vi "Setup Motors.vi"   [LabVIEW 2014]
uses:
  <vilib>/Rock Robotics/SystemInterfaces/DIO/FPGA_DIOPWMChannel.ctl
  <vilib>/Rock Robotics/WPI/Joystick/WPI_JoystickDeviceEnum.ctl
  <vilib>/Rock Robotics/SystemInterfaces/Typedef/FPGA_TypedefDigitalModule.ctl
  <vilib>/Rock Robotics/SystemInterfaces/Typedef/FPGA_TypedefAnalogModule.ctl
  <vilib>/Rock Robotics/SystemInterfaces/AI/FPGA_AIChannel.ctl
  <vilib>/Rock Robotics/WPI/SafetyOutput/WPI_SafetyOutputConfigMenu.ctl
  <vilib>/Rock Robotics/WPI/Solenoid/WPI_SolenoidChannel.ctl
  <vilib>/Rock Robotics/SystemInterfaces/AI/FPGA_AIGyroChannel.ctl
  <vilib>/Rock Robotics/SystemInterfaces/Typedef/FPGA_TypedefAnalogModuleForGyro.ctl
  <vilib>/Rock Robotics/SystemInterfaces/DIO/FPGA_DIOChannel.ctl
  NavX Code/navX-MXP Library/COMMON/TypeDefs/Value TypeDefs/navX Interface Protocol.ctl
  <vilib>/Rock Robotics/SystemInterfaces/spilib/spi_bus.ctl
  <vilib>/Rock Robotics/SystemInterfaces/i2clib/i2c_bus.ctl
  NavX Code/navX-MXP Library/COMMON/TypeDefs/Value TypeDefs/navX Update Rate.ctl
  <vilib>/Rock Robotics/WPI/MotorControl/WPI_MotorControlOpen Jaguar.vi
  <vilib>/Rock Robotics/WPI/MotorControl/WPI_MotorControlOpen Talon.vi
  <vilib>/Rock Robotics/WPI/Solenoid/WPI_SolenoidOpenSingle.vi
  <vilib>/Rock Robotics/WPI/Switch/WPI_SwitchOpenLimit.vi
  <vilib>/Rock Robotics/WPI/Counter/WPI_CounterDigitalInputToDigitalSource.vi
  <vilib>/Rock Robotics/WPI/Counter/WPI_CounterOpen UpDown Mode.vi
  Global Variables.vi
  NavX Code/navX-MXP Library/navX-MXP IMU.lvlib
types:
  T1 = typedef "FPGA_DIOChannel.ctl" = enum8{"DIO 0", "DIO 1", "DIO 2", "DIO 3", "DIO 4", "DIO 5", "DIO 6", "DIO 7", "DIO 8", "DIO 9", "DIO MXP 0", "DIO MXP 1", "DIO MXP 2", "DIO MXP 3", "DIO MXP 4", "DIO MXP 5", "DIO MXP 6", "DIO MXP 7", "DIO MXP 8", "DIO MXP 9", "DIO MXP 10", "DIO MXP 11", "DIO MXP 12", "DIO MXP 13", "DIO MXP 14", "DIO MXP 15", "Invalid"}
  T2 = typedef "navX-MXP IMU.lvlib/navX Update Rate.ctl" = u8
  T3 = typedef "i2c_bus.ctl" = enum16{"I2C On-Board", "I2C MXP", "Invalid"}
  T4 = typedef "spi_bus.ctl" = enum16{"SPI On-Board, CS0", "SPI On-Board, CS1", "SPI On-Board, CS2", "SPI On-Board, CS3", "SPI MXP", "Invalid"}
  T5 = typedef "navX-MXP IMU.lvlib/navX Interface Protocol.ctl" = enum16{"SPI", "I2C"}
  T6 = typedef "WPI_SafetyOutputConfigMenu.ctl" = enum16{"Enable", "Disable"}
  T7 = typedef "FPGA_TypedefDigitalModule.ctl" = enum16{"Controller 1"}
  T8 = typedef "FPGA_TypedefAnalogModuleForGyro.ctl" = enum16{"Controller 1"}
  T9 = typedef "FPGA_AIGyroChannel.ctl" = enum8{"AI 0", "AI 1", "Invalid"}
  T10 = typedef "WPI_SolenoidChannel.ctl" = enum8{"Solenoid 0", "Solenoid 1", "Solenoid 2", "Solenoid 3", "Solenoid 4", "Solenoid 5", "Solenoid 6", "Solenoid 7", "Invalid"}
  T11 = typedef "FPGA_DIOPWMChannel.ctl" = enum8{"PWM 0", "PWM 1", "PWM 2", "PWM 3", "PWM 4", "PWM 5", "PWM 6", "PWM 7", "PWM 8", "PWM 9", "PWM MXP 0", "PWM MXP 1", "PWM MXP 2", "PWM MXP 3", "PWM MXP 4", "PWM MXP 5", "PWM MXP 6", "PWM MXP 7", "PWM MXP 8", "PWM MXP 9", "Invalid"}
  T12 = typedef "FPGA_AIChannel.ctl" = enum8{"AI 0", "AI 1", "AI 2", "AI 3", "AI MXP 0", "AI MXP 1", "AI MXP 2", "AI MXP 3", "Invalid"}
  T13 = typedef "FPGA_TypedefAnalogModule.ctl" = enum16{"Controller 1"}
  T14 = typedef "WPI_JoystickDeviceEnum.ctl" = enum16{"USB 0", "USB 1", "USB 2", "USB 3", "USB 4", "USB 5"}
  T15 = typedef "WPI_MotorControlDeviceRef.ctl" = cluster{"DeviceStatus":errorcluster, "Type":T16, "PWM":cluster{"Controller":T7, "PWM Channel":T11, "DeadBand":T17}, "CAN":cluster{"Device Number":u8, "Control Mode":T18, "Semaphore":T19, "Max Vout":dbl, "TalonSRX Control Mode":T20}, "Invert":bool, "TransformRef":T21, "InvTransformRef":T21}
  T16 = typedef "WPI_MotorControlType.ctl" = enum16{"PWM", "CAN", "CANTalonSRX"}
  T17 = typedef "WPI_PWMDeadband.ctl" = cluster{"Name":string, "maxPositivePwm":i32, "minPositivePwm":i32, "centerPwm":i32, "maxNegativePwm":i32, "minNegativePwm":i32, "angularRange":u16}
  T18 = typedef "WPI_CANJaguar_ControlMode.ctl" = enum8{"Percent VBus", "Current", "Speed", "Position", "Voltage"}
  T19 = typedef "Semaphore RefNum" = refnum<k1>
  T20 = typedef "WPI_CANTalonSRX_APIControlMode.ctl" = enum8{"Percent VBus", "Speed", "Position", "Slave", "Unchanged / Invalid"}
  T21 = typedef "WPI_PWMTransform_ConPane.ctl" = refnum<vi>
  T22 = typedef "WPI_GyroDevRef.ctl" = cluster{"DevStatus":errorcluster, "Analog Module":T13, "Analog Channel":T12, "Offset":dbl, "Gain (VoltsPerDegree/Second)":dbl}
  T23 = typedef "WPI_SolenoidDevRef.ctl" = cluster{"DevStatus":errorcluster, "Pneumatics Control Module":u8, "Forward Solenoid Channel":T10, "Reverse Solenoid Channel":T10}
  T24 = typedef "WPI_SwitchDevRef.ctl" = cluster{"DevStatus":errorcluster, "DIO Channel":T1, "Controller":T7, "CntIndex":T25, "Normally Closed":bool}
  T25 = typedef "FPGA_CounterCtrSystemIndex.ctl" = enum8{"Ctr 0", "Ctr 1", "Ctr 2", "Ctr 3", "Ctr 4", "Ctr 5", "Ctr 6", "Ctr 7", "Invalid"}
  T26 = typedef "WPI_AnalogChannelDevRef.ctl" = cluster{"DevStatus":errorcluster, "Controller":T13, "Analog Channel":T12}
  T27 = typedef "WPI_DigitalInputDevRef.ctl" = cluster{"DevStatus":errorcluster, "DIO Channel":T1, "Controller":T7}
  T28 = typedef "FPGA_CounterEncoderSourceConvertionLVSourceType.ctl" = cluster{"DevStatus":errorcluster, "AnalogTriggerMode?":bool, "DigitalMode":cluster{"Controller":T7, "DIO Channel":T29}, "AnalogTriggerMode":cluster{"AnalogTriggerIndex":T30, "OutputType":T31}}
  T29 = typedef "FPGA_DIODigitalSourceChannel.ctl" = enum8{"DIO 0", "DIO 1", "DIO 2", "DIO 3", "DIO 4", "DIO 5", "DIO 6", "DIO 7", "DIO 8", "DIO 9", "DIO MXP 0", "DIO MXP 1", "DIO MXP 2", "DIO MXP 3", "DIO MXP 4", "DIO MXP 5", "DIO MXP 6", "DIO MXP 7", "DIO MXP 8", "DIO MXP 9", "DIO MXP 10", "DIO MXP 11", "DIO MXP 12", "DIO MXP 13", "DIO MXP 14", "DIO MXP 15", "Disabled"}
  T30 = typedef "FPGA_AnalogTriggerIndex.ctl" = enum8{"Trig 0", "Trig 1", "Trig 2", "Trig 3", "Trig 4", "Trig 5", "Trig 6", "Trig 7", "Invalid"}
  T31 = typedef "FPGA_AnalogTriggerOutType.ctl" = enum16{"InWindow", "TriggerState", "Rising", "Falling"}
  T32 = typedef "WPI_EncoderDevRef.ctl" = cluster{"DevStatus":errorcluster, "EncoderIndex":T33, "CounterIndex":T25, "DistancePerCount":dbl, "Decoding Type":T34}
  T33 = typedef "FPGA_EncoderIdx.ctl" = enum8{"Enc 0", "Enc 1", "Enc 2", "Enc 3", "Enc 4", "Enc 5", "Enc 6", "Enc 7", "Invalid"}
  T34 = typedef "WPI_EncoderType.ctl" = enum16{"1x", "2x", "4x"}
  T35 = typedef "WPI_CounterDevRef.ctl" = cluster{"DevStatus":errorcluster, "CntIndex":T25}
  T36 = typedef "navX-MXP IMU.lvlib/navX Device TypeDef.ctl" = cluster{"navX Interface Protocol":T5, "navX Interface Protocol TypeDefs":cluster{"SPIDevRef":T37, "I2CDevRef":T38}, "navX System Information":cluster{"Board Information":T39, "Status":T40, "Offsets":T44}, "navX Common Information":cluster{"Update Rate (4Hz-60Hz)":T2, "refnum name":string, "error":errorcluster}}
  T37 = typedef "WPI_SPIDevRef.ctl" = cluster{"DevStatus":errorcluster, "Handle":i32, "Controller":T7, "SPI Bus":T4}
  T38 = typedef "WPI_I2CDevRef.ctl" = cluster{"DevStatus":errorcluster, "Controller":T7, "Device Address":u8, "Handle":i32, "I2C Bus":T3}
  T39 = typedef "navX-MXP IMU.lvlib/navX Board Information.ctl" = cluster{"WhoAmI (50 | 0x32)":u8, "Board Revision":u8, "Firmware Major Version":u8, "Firmware Minor Version":u8}
  T40 = typedef "navX-MXP IMU.lvlib/navX Status Data.ctl" = cluster{"Update Rate Hz":u8, "Accelerometer Full-Scale Range":u8, "Gyro Full-Scale Range":u16, "NAVX_OP_STATUS":T41, "NAVX_CAL_STATUS":T42, "NAVX_SELFTEST_STATUS":u8, "NAVX_SENSOR_STATUS":T43}
  T41 = typedef "navX-MXP IMU.lvlib/navX NAVX_OP_STATUS.ctl" = u8
  T42 = typedef "navX-MXP IMU.lvlib/navX NAVX_CAL_STATUS.ctl" = u8
  T43 = typedef "navX-MXP IMU.lvlib/navX NAVX_SENSOR_STATUS.ctl" = cluster{"MOVING":bool, "YAW_STABLE":bool, "MAG_DISTURBANCE":bool, "ALTITUDE_VALID":bool, "SEALEVEL_PRESS_SET":bool, "FUSED_HEADING_VALID":bool}
  T44 = typedef "navX-MXP IMU.lvlib/navX Offsets Data.ctl" = cluster{"Yaw":dbl, "Quat W":dbl, "Quat X":dbl, "Quat Y":dbl, "Quat Z":dbl}
  T45 = typedef "WPI_JoystickDevRef.ctl" = cluster{"Device":T14}
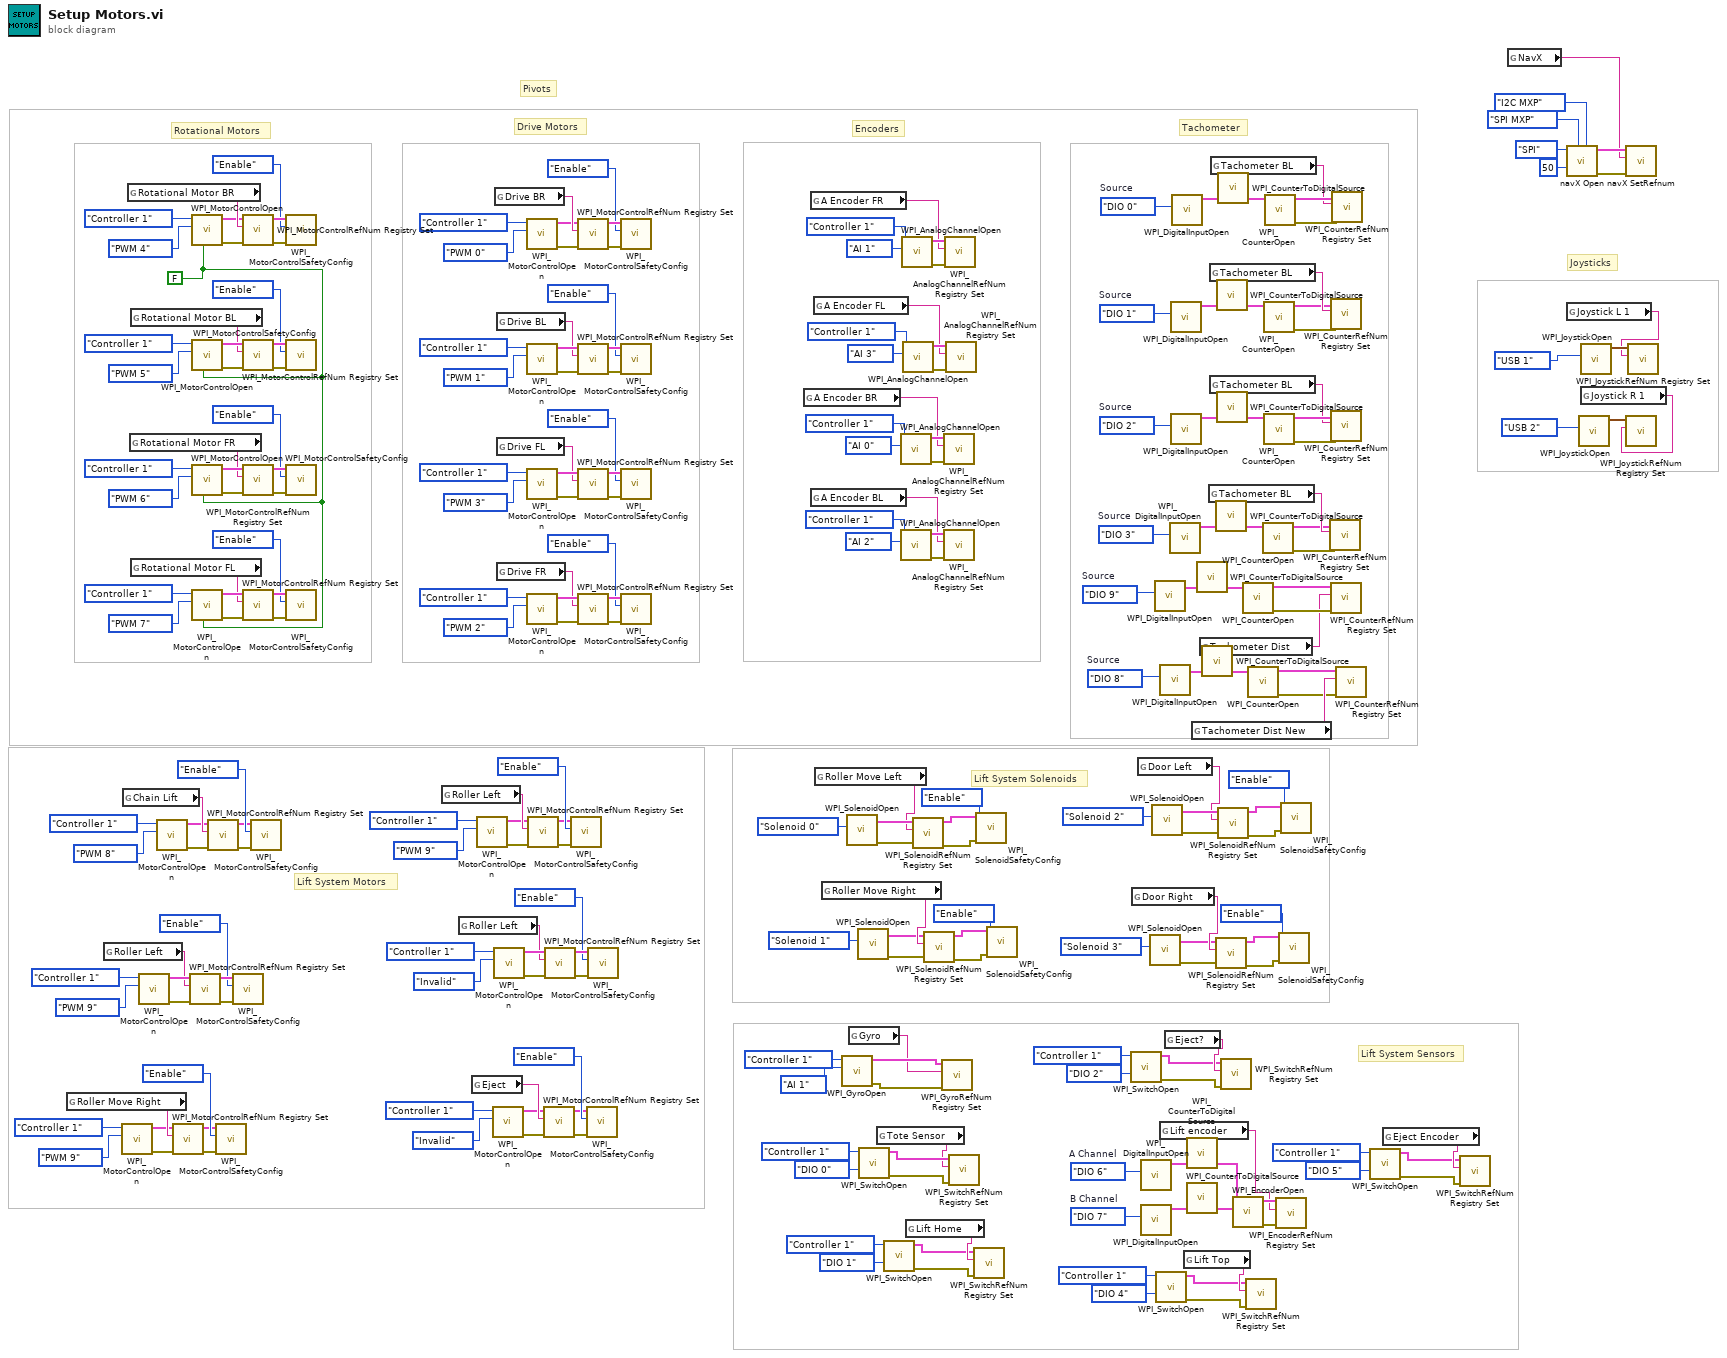
[diagram p0: block diagram]
diagram:
  w4 = FPGA_DIOChannel."DIO 8"  # Source
  w9 = FPGA_DIOChannel."DIO 9"  # Source
  w21 = FPGA_DIOChannel."DIO 3"  # Source
  w30 = FPGA_DIOChannel."DIO 2"  # Source
  w33 = FPGA_DIOChannel."DIO 1"  # Source
  w42 = FPGA_DIOChannel."DIO 0"  # Source
  w44 = FALSE ("Invert")
  w53 = FPGA_DIOChannel."DIO 7"  # B Channel
  w52 = FPGA_DIOChannel."DIO 6"  # A Channel
  # "Tachometer"
  # "Lift System Sensors"
  # "Lift System Solenoids"
  # "Lift System Motors"
  # "Encoders"
  # "Joysticks"
  # "Pivots"
  # "Rotational Motors"
  # "Drive Motors"
  n1 = global read "Global Variables.vi" "Roller Move Right"() -> (w142:string)
  n2 = global read "Global Variables.vi" "Roller Left"() -> (w145:string)
  n3 = call-poly <vilib>:"WPI_MotorControlOpen.vi"("PWM Channel"=FPGA_DIOPWMChannel."PWM 9", "Controller"=FPGA_TypedefDigitalModule."Controller 1") -> ("error out"=w137:errorcluster, "MotorControlDeviceRef"=w136:T15)  [unwired: 8 in]
  n4 = global read "Global Variables.vi" "Chain Lift"() -> (w158:string)
  n5 = global read "Global Variables.vi" "Rotational Motor BR"() -> (w212:string)
  n6 = global read "Global Variables.vi" "Rotational Motor FR"() -> (w186:string)
  n7 = global read "Global Variables.vi" "Rotational Motor BL"() -> (w187:string)
  n8 = global read "Global Variables.vi" "Rotational Motor FL"() -> (w185:string)
  n9 = call-poly <vilib>:"WPI_MotorControlOpen.vi"("PWM Channel"=FPGA_DIOPWMChannel."PWM 9", "Controller"=FPGA_TypedefDigitalModule."Controller 1") -> ("error out"=w150:errorcluster, "MotorControlDeviceRef"=w151:T15)  [unwired: 8 in]
  n10 = call-poly <vilib>:"WPI_MotorControlOpen.vi"("PWM Channel"=FPGA_DIOPWMChannel."PWM 8", "Controller"=FPGA_TypedefDigitalModule."Controller 1") -> ("error out"=w153:errorcluster, "MotorControlDeviceRef"=w152:T15)  [unwired: 8 in]
  n11 = call <vilib>:"WPI_MotorControlRefNum Registry Set.vi"("error in (no error)"=w137, "refnum name"=w142, "MotorControlDevRef"=w136) -> ("error out"=w139:errorcluster, "MotorControlDevRef"=w138:T15)  [unwired: 7 in]
  n12 = call <vilib>:"WPI_MotorControlRefNum Registry Set.vi"("error in (no error)"=w150, "refnum name"=w145, "MotorControlDevRef"=w151) -> ("error out"=w148:errorcluster, "MotorControlDevRef"=w149:T15)  [unwired: 7 in]
  n13 = call-poly <vilib>:"WPI_MotorControlOpen.vi"("Invert"=w44, "PWM Channel"=FPGA_DIOPWMChannel."PWM 4", "Controller"=FPGA_TypedefDigitalModule."Controller 1") -> ("error out"=w210:errorcluster, "MotorControlDeviceRef"=w211:T15)  [unwired: 7 in]
  n14 = call-poly <vilib>:"WPI_MotorControlOpen.vi"("Invert"=w44, "PWM Channel"=FPGA_DIOPWMChannel."PWM 5", "Controller"=FPGA_TypedefDigitalModule."Controller 1") -> ("error out"=w204:errorcluster, "MotorControlDeviceRef"=w205:T15)  [unwired: 7 in]
  n15 = call-poly <vilib>:"WPI_MotorControlOpen.vi"("Invert"=w44, "PWM Channel"=FPGA_DIOPWMChannel."PWM 6", "Controller"=FPGA_TypedefDigitalModule."Controller 1") -> ("error out"=w198:errorcluster, "MotorControlDeviceRef"=w199:T15)  [unwired: 7 in]
  n16 = call-poly <vilib>:"WPI_MotorControlOpen.vi"("Invert"=w44, "PWM Channel"=FPGA_DIOPWMChannel."PWM 7", "Controller"=FPGA_TypedefDigitalModule."Controller 1") -> ("error out"=w192:errorcluster, "MotorControlDeviceRef"=w193:T15)  [unwired: 7 in]
  n17 = call <vilib>:"WPI_MotorControlRefNum Registry Set.vi"("error in (no error)"=w153, "refnum name"=w158, "MotorControlDevRef"=w152) -> ("error out"=w155:errorcluster, "MotorControlDevRef"=w154:T15)  [unwired: 7 in]
  n18 = call <vilib>:"WPI_MotorControlSafetyConfig.vi"("error in (no error)"=w139, "mode"=WPI_SafetyOutputConfigMenu."Enable", "MotorControlDevRef"=w138) -> ()  [unwired: 7 in, 2 out]
  n19 = call <vilib>:"WPI_MotorControlSafetyConfig.vi"("error in (no error)"=w148, "mode"=WPI_SafetyOutputConfigMenu."Enable", "MotorControlDevRef"=w149) -> ()  [unwired: 7 in, 2 out]
  n20 = call <vilib>:"WPI_MotorControlRefNum Registry Set.vi"("error in (no error)"=w210, "refnum name"=w212, "MotorControlDevRef"=w211) -> ("error out"=w208:errorcluster, "MotorControlDevRef"=w209:T15)  [unwired: 7 in]
  n21 = call <vilib>:"WPI_MotorControlRefNum Registry Set.vi"("error in (no error)"=w204, "refnum name"=w187, "MotorControlDevRef"=w205) -> ("error out"=w202:errorcluster, "MotorControlDevRef"=w203:T15)  [unwired: 7 in]
  n22 = call <vilib>:"WPI_MotorControlRefNum Registry Set.vi"("error in (no error)"=w198, "refnum name"=w186, "MotorControlDevRef"=w199) -> ("error out"=w196:errorcluster, "MotorControlDevRef"=w197:T15)  [unwired: 7 in]
  n23 = call <vilib>:"WPI_MotorControlRefNum Registry Set.vi"("error in (no error)"=w192, "refnum name"=w185, "MotorControlDevRef"=w193) -> ("error out"=w190:errorcluster, "MotorControlDevRef"=w191:T15)  [unwired: 7 in]
  n24 = call <vilib>:"WPI_MotorControlSafetyConfig.vi"("error in (no error)"=w155, "mode"=WPI_SafetyOutputConfigMenu."Enable", "MotorControlDevRef"=w154) -> ()  [unwired: 7 in, 2 out]
  n25 = call <vilib>:"WPI_MotorControlSafetyConfig.vi"("error in (no error)"=w208, "mode"=WPI_SafetyOutputConfigMenu."Enable", "MotorControlDevRef"=w209) -> ()  [unwired: 7 in, 2 out]
  n26 = call <vilib>:"WPI_MotorControlSafetyConfig.vi"("error in (no error)"=w202, "mode"=WPI_SafetyOutputConfigMenu."Enable", "MotorControlDevRef"=w203) -> ()  [unwired: 7 in, 2 out]
  n27 = call <vilib>:"WPI_MotorControlSafetyConfig.vi"("error in (no error)"=w196, "mode"=WPI_SafetyOutputConfigMenu."Enable", "MotorControlDevRef"=w197) -> ()  [unwired: 7 in, 2 out]
  n28 = call <vilib>:"WPI_MotorControlSafetyConfig.vi"("error in (no error)"=w190, "mode"=WPI_SafetyOutputConfigMenu."Enable", "MotorControlDevRef"=w191) -> ()  [unwired: 7 in, 2 out]
  n29 = global read "Global Variables.vi" "Roller Left"() -> (w134:string)
  n30 = global read "Global Variables.vi" "Roller Left"() -> (w121:string)
  n31 = global read "Global Variables.vi" "Eject"() -> (w118:string)
  n32 = call-poly <vilib>:"WPI_MotorControlOpen.vi"("PWM Channel"=FPGA_DIOPWMChannel."PWM 9", "Controller"=FPGA_TypedefDigitalModule."Controller 1") -> ("error out"=w129:errorcluster, "MotorControlDeviceRef"=w128:T15)  [unwired: 8 in]
  n33 = call-poly <vilib>:"WPI_MotorControlOpen.vi"("PWM Channel"=FPGA_DIOPWMChannel."Invalid", "Controller"=FPGA_TypedefDigitalModule."Controller 1") -> ("error out"=w113:errorcluster, "MotorControlDeviceRef"=w112:T15)  [unwired: 8 in]
  n34 = call-poly <vilib>:"WPI_MotorControlOpen.vi"("PWM Channel"=FPGA_DIOPWMChannel."Invalid", "Controller"=FPGA_TypedefDigitalModule."Controller 1") -> ("error out"=w126:errorcluster, "MotorControlDeviceRef"=w127:T15)  [unwired: 8 in]
  n35 = global read "Global Variables.vi" "Drive BR"() -> (w249:string)
  n36 = global read "Global Variables.vi" "Drive BL"() -> (w224:string)
  n37 = global read "Global Variables.vi" "Drive FL"() -> (w223:string)
  n38 = global read "Global Variables.vi" "Drive FR"() -> (w222:string)
  n39 = call-poly <vilib>:"WPI_MotorControlOpen.vi"("PWM Channel"=FPGA_DIOPWMChannel."PWM 0", "Controller"=FPGA_TypedefDigitalModule."Controller 1") -> ("error out"=w247:errorcluster, "MotorControlDeviceRef"=w248:T15)  [unwired: 8 in]
  n40 = call-poly <vilib>:"WPI_MotorControlOpen.vi"("PWM Channel"=FPGA_DIOPWMChannel."PWM 1", "Controller"=FPGA_TypedefDigitalModule."Controller 1") -> ("error out"=w241:errorcluster, "MotorControlDeviceRef"=w242:T15)  [unwired: 8 in]
  n41 = call-poly <vilib>:"WPI_MotorControlOpen.vi"("PWM Channel"=FPGA_DIOPWMChannel."PWM 3", "Controller"=FPGA_TypedefDigitalModule."Controller 1") -> ("error out"=w235:errorcluster, "MotorControlDeviceRef"=w236:T15)  [unwired: 8 in]
  n42 = call-poly <vilib>:"WPI_MotorControlOpen.vi"("PWM Channel"=FPGA_DIOPWMChannel."PWM 2", "Controller"=FPGA_TypedefDigitalModule."Controller 1") -> ("error out"=w229:errorcluster, "MotorControlDeviceRef"=w230:T15)  [unwired: 8 in]
  n43 = call <vilib>:"WPI_MotorControlRefNum Registry Set.vi"("error in (no error)"=w129, "refnum name"=w134, "MotorControlDevRef"=w128) -> ("error out"=w131:errorcluster, "MotorControlDevRef"=w130:T15)  [unwired: 7 in]
  n44 = call <vilib>:"WPI_MotorControlRefNum Registry Set.vi"("error in (no error)"=w113, "refnum name"=w118, "MotorControlDevRef"=w112) -> ("error out"=w115:errorcluster, "MotorControlDevRef"=w114:T15)  [unwired: 7 in]
  n45 = call <vilib>:"WPI_MotorControlRefNum Registry Set.vi"("error in (no error)"=w126, "refnum name"=w121, "MotorControlDevRef"=w127) -> ("error out"=w124:errorcluster, "MotorControlDevRef"=w125:T15)  [unwired: 7 in]
  n46 = call <vilib>:"WPI_MotorControlSafetyConfig.vi"("error in (no error)"=w131, "mode"=WPI_SafetyOutputConfigMenu."Enable", "MotorControlDevRef"=w130) -> ()  [unwired: 7 in, 2 out]
  n47 = call <vilib>:"WPI_MotorControlRefNum Registry Set.vi"("error in (no error)"=w247, "refnum name"=w249, "MotorControlDevRef"=w248) -> ("error out"=w245:errorcluster, "MotorControlDevRef"=w246:T15)  [unwired: 7 in]
  n48 = call <vilib>:"WPI_MotorControlRefNum Registry Set.vi"("error in (no error)"=w241, "refnum name"=w224, "MotorControlDevRef"=w242) -> ("error out"=w239:errorcluster, "MotorControlDevRef"=w240:T15)  [unwired: 7 in]
  n49 = call <vilib>:"WPI_MotorControlRefNum Registry Set.vi"("error in (no error)"=w235, "refnum name"=w223, "MotorControlDevRef"=w236) -> ("error out"=w233:errorcluster, "MotorControlDevRef"=w234:T15)  [unwired: 7 in]
  n50 = call <vilib>:"WPI_MotorControlRefNum Registry Set.vi"("error in (no error)"=w229, "refnum name"=w222, "MotorControlDevRef"=w230) -> ("error out"=w227:errorcluster, "MotorControlDevRef"=w228:T15)  [unwired: 7 in]
  n51 = call <vilib>:"WPI_MotorControlSafetyConfig.vi"("error in (no error)"=w115, "mode"=WPI_SafetyOutputConfigMenu."Enable", "MotorControlDevRef"=w114) -> ()  [unwired: 7 in, 2 out]
  n52 = call <vilib>:"WPI_MotorControlSafetyConfig.vi"("error in (no error)"=w124, "mode"=WPI_SafetyOutputConfigMenu."Enable", "MotorControlDevRef"=w125) -> ()  [unwired: 7 in, 2 out]
  n53 = call <vilib>:"WPI_MotorControlSafetyConfig.vi"("error in (no error)"=w245, "mode"=WPI_SafetyOutputConfigMenu."Enable", "MotorControlDevRef"=w246) -> ()  [unwired: 7 in, 2 out]
  n54 = call <vilib>:"WPI_MotorControlSafetyConfig.vi"("error in (no error)"=w239, "mode"=WPI_SafetyOutputConfigMenu."Enable", "MotorControlDevRef"=w240) -> ()  [unwired: 7 in, 2 out]
  n55 = call <vilib>:"WPI_MotorControlSafetyConfig.vi"("error in (no error)"=w233, "mode"=WPI_SafetyOutputConfigMenu."Enable", "MotorControlDevRef"=w234) -> ()  [unwired: 7 in, 2 out]
  n56 = call <vilib>:"WPI_MotorControlSafetyConfig.vi"("error in (no error)"=w227, "mode"=WPI_SafetyOutputConfigMenu."Enable", "MotorControlDevRef"=w228) -> ()  [unwired: 7 in, 2 out]
  n57 = global read "Global Variables.vi" "A Encoder BR"() -> (w161:string)
  n58 = global read "Global Variables.vi" "A Encoder FR"() -> (w163:string)
  n59 = global read "Global Variables.vi" "A Encoder BL"() -> (w162:string)
  n60 = global read "Global Variables.vi" "A Encoder FL"() -> (w160:string)
  n61 = global read "Global Variables.vi" "Roller Move Left"() -> (w106:string)
  n62 = global read "Global Variables.vi" "Roller Move Right"() -> (w105:string)
  n63 = call <vilib>:"WPI_GyroOpen.vi"("Analog Channel"=FPGA_AIGyroChannel."AI 1", "Controller"=FPGA_TypedefAnalogModuleForGyro."Controller 1") -> ("error out"=w86:errorcluster, "GyroDevRef"=w87:T22)  [unwired: 7 in, 1 out]
  n64 = call-poly <vilib>:"WPI_SolenoidOpen.vi"("Solenoid Channel"=WPI_SolenoidChannel."Solenoid 0") -> ("error out"=w108:errorcluster, "SolenoidDevRef"=w109:T23)  [unwired: 9 in]
  n65 = global read "Global Variables.vi" "Gyro"() -> (w83:string)
  n66 = call-poly <vilib>:"WPI_SolenoidOpen.vi"("Solenoid Channel"=WPI_SolenoidChannel."Solenoid 1") -> ("error out"=w103:errorcluster, "SolenoidDevRef"=w102:T23)  [unwired: 9 in]
  n67 = call-poly <vilib>:"WPI_SwitchOpen.vi"("DIO Channel"=FPGA_DIOChannel."DIO 0", "Controller"=FPGA_TypedefDigitalModule."Controller 1") -> ("error out"=w81:errorcluster, "SwitchDevRef"=w82:T24)  [unwired: 8 in]
  n68 = global read "Global Variables.vi" "Tote Sensor"() -> (w78:string)
  n69 = call-poly <vilib>:"WPI_SwitchOpen.vi"("DIO Channel"=FPGA_DIOChannel."DIO 1", "Controller"=FPGA_TypedefDigitalModule."Controller 1") -> ("error out"=w74:errorcluster, "SwitchDevRef"=w73:T24)  [unwired: 8 in]
  n70 = call <vilib>:"WPI_AnalogChannelOpen.vi"("Analog Channel"=FPGA_AIChannel."AI 0", "Controller"=FPGA_TypedefAnalogModule."Controller 1") -> ("error out"=w170:errorcluster, "AIDeviceRef"=w171:T26)  [unwired: 8 in]
  n71 = call <vilib>:"WPI_AnalogChannelOpen.vi"("Analog Channel"=FPGA_AIChannel."AI 2", "Controller"=FPGA_TypedefAnalogModule."Controller 1") -> ("error out"=w166:errorcluster, "AIDeviceRef"=w167:T26)  [unwired: 8 in]
  n72 = call <vilib>:"WPI_AnalogChannelOpen.vi"("Analog Channel"=FPGA_AIChannel."AI 1", "Controller"=FPGA_TypedefAnalogModule."Controller 1") -> ("error out"=w178:errorcluster, "AIDeviceRef"=w179:T26)  [unwired: 8 in]
  n73 = call <vilib>:"WPI_AnalogChannelOpen.vi"("Analog Channel"=FPGA_AIChannel."AI 3", "Controller"=FPGA_TypedefAnalogModule."Controller 1") -> ("error out"=w174:errorcluster, "AIDeviceRef"=w175:T26)  [unwired: 8 in]
  n74 = global read "Global Variables.vi" "Lift Home"() -> (w77:string)
  n75 = call <vilib>:"WPI_SolenoidRefNum Registry Set.vi"("error in (no error)"=w108, "refnum name"=w106, "SolenoidDevRef"=w109) -> ("error out"=w110:errorcluster, "SolenoidDevRef"=w111:T23)  [unwired: 7 in]
  n76 = call <vilib>:"WPI_SolenoidRefNum Registry Set.vi"("error in (no error)"=w103, "refnum name"=w105, "SolenoidDevRef"=w102) -> ("error out"=w101:errorcluster, "SolenoidDevRef"=w100:T23)  [unwired: 7 in]
  n77 = call <vilib>:"WPI_GyroRefNum Registry Set.vi"("error in (no error)"=w86, "refnum name"=w83, "GyroDevRef"=w87) -> ()  [unwired: 7 in, 2 out]
  n78 = call <vilib>:"WPI_AnalogChannelRefNum Registry Set.vi"("error in (no error)"=w170, "refnum name"=w161, "AIDeviceRef"=w171) -> ()  [unwired: 7 in, 2 out]
  n79 = call <vilib>:"WPI_AnalogChannelRefNum Registry Set.vi"("error in (no error)"=w166, "refnum name"=w162, "AIDeviceRef"=w167) -> ()  [unwired: 7 in, 2 out]
  n80 = call <vilib>:"WPI_AnalogChannelRefNum Registry Set.vi"("error in (no error)"=w178, "refnum name"=w163, "AIDeviceRef"=w179) -> ()  [unwired: 7 in, 2 out]
  n81 = call <vilib>:"WPI_AnalogChannelRefNum Registry Set.vi"("error in (no error)"=w174, "refnum name"=w160, "AIDeviceRef"=w175) -> ()  [unwired: 7 in, 2 out]
  n82 = call <vilib>:"WPI_SwitchRefNum Registry Set.vi"("error in (no error)"=w81, "refnum name"=w78, "SwitchDevRef"=w82) -> ()  [unwired: 7 in, 2 out]
  n83 = call <vilib>:"WPI_SwitchRefNum Registry Set.vi"("error in (no error)"=w74, "refnum name"=w77, "SwitchDevRef"=w73) -> ()  [unwired: 7 in, 2 out]
  n84 = call <vilib>:"WPI_SolenoidSafetyConfig.vi"("error in (no error)"=w110, "mode"=WPI_SafetyOutputConfigMenu."Enable", "SolenoidDevRef"=w111) -> ()  [unwired: 7 in, 2 out]
  n85 = call <vilib>:"WPI_SolenoidSafetyConfig.vi"("error in (no error)"=w101, "mode"=WPI_SafetyOutputConfigMenu."Enable", "SolenoidDevRef"=w100) -> ()  [unwired: 7 in, 2 out]
  n86 = call-poly <vilib>:"WPI_SwitchOpen.vi"("DIO Channel"=FPGA_DIOChannel."DIO 2", "Controller"=FPGA_TypedefDigitalModule."Controller 1") -> ("error out"=w64:errorcluster, "SwitchDevRef"=w63:T24)  [unwired: 8 in]
  n87 = global read "Global Variables.vi" "Door Right"() -> (w93:string)
  n88 = global read "Global Variables.vi" "Door Left"() -> (w94:string)
  n89 = call <vilib>:"WPI_DigitalInputOpen.vi"("DIO Channel"=w52) -> ("DigitalInputDevRef"=w49:T27)  [unwired: 2 in, 8 out]
  n90 = call <vilib>:"WPI_DigitalInputOpen.vi"("DIO Channel"=w53) -> ("DigitalInputDevRef"=w50:T27)  [unwired: 2 in, 8 out]
  n91 = call-poly <vilib>:"WPI_SolenoidOpen.vi"("Solenoid Channel"=WPI_SolenoidChannel."Solenoid 3") -> ("error out"=w91:errorcluster, "SolenoidDevRef"=w90:T23)  [unwired: 9 in]
  n92 = call-poly <vilib>:"WPI_SolenoidOpen.vi"("Solenoid Channel"=WPI_SolenoidChannel."Solenoid 2") -> ("error out"=w96:errorcluster, "SolenoidDevRef"=w97:T23)  [unwired: 9 in]
  n93 = call <vilib>:"WPI_DigitalInputOpen.vi"("DIO Channel"=w9) -> ("DigitalInputDevRef"=w12:T27)  [unwired: 2 in, 8 out]
  n94 = call-poly <vilib>:"WPI_SwitchOpen.vi"("DIO Channel"=FPGA_DIOChannel."DIO 4", "Controller"=FPGA_TypedefDigitalModule."Controller 1") -> ("error out"=w69:errorcluster, "SwitchDevRef"=w68:T24)  [unwired: 8 in]
  n95 = call <vilib>:"WPI_DigitalInputOpen.vi"("DIO Channel"=w4) -> ("DigitalInputDevRef"=w1:T27)  [unwired: 2 in, 8 out]
  n96 = global read "Global Variables.vi" "Lift encoder"() -> (w45:string)
  n97 = global read "Global Variables.vi" "Eject?"() -> (w67:string)
  n98 = call <vilib>:"WPI_DigitalInputOpen.vi"("DIO Channel"=w21) -> ("DigitalInputDevRef"=w22:T27)  [unwired: 2 in, 8 out]
  n99 = call <vilib>:"WPI_DigitalInputOpen.vi"("DIO Channel"=w33) -> ("DigitalInputDevRef"=w34:T27)  [unwired: 2 in, 8 out]
  n100 = call <vilib>:"WPI_DigitalInputOpen.vi"("DIO Channel"=w30) -> ("DigitalInputDevRef"=w29:T27)  [unwired: 2 in, 8 out]
  n101 = call <vilib>:"WPI_DigitalInputOpen.vi"("DIO Channel"=w42) -> ("DigitalInputDevRef"=w41:T27)  [unwired: 2 in, 8 out]
  n102 = global read "Global Variables.vi" "Lift Top"() -> (w72:string)
  n103 = call-poly <vilib>:"WPI_CounterToDigitalSource.vi"("DigitalInputDevRef"=w49) -> ("Digital Source"=w48:T28)  [unwired: 6 out]
  n104 = call-poly <vilib>:"WPI_CounterToDigitalSource.vi"("DigitalInputDevRef"=w50) -> ("Digital Source"=w51:T28)  [unwired: 6 out]
  n105 = global read "Global Variables.vi" "Tachometer Dist New"() -> (w6:string)
  n106 = call-poly <vilib>:"WPI_CounterToDigitalSource.vi"("DigitalInputDevRef"=w12) -> ("Digital Source"=w11:T28)  [unwired: 6 out]
  n107 = global read "Global Variables.vi" "Tachometer Dist"() -> (w7:string)
  n108 = call-poly <vilib>:"WPI_CounterToDigitalSource.vi"("DigitalInputDevRef"=w1) -> ("Digital Source"=w2:T28)  [unwired: 6 out]
  n109 = global read "Global Variables.vi" "Tachometer BL"() -> (w25:string)
  n110 = global read "Global Variables.vi" "Tachometer BL"() -> (w37:string)
  n111 = global read "Global Variables.vi" "Tachometer BL"() -> (w26:string)
  n112 = global read "Global Variables.vi" "Tachometer BL"() -> (w38:string)
  n113 = call-poly <vilib>:"WPI_CounterToDigitalSource.vi"("DigitalInputDevRef"=w22) -> ("Digital Source"=w20:T28)  [unwired: 6 out]
  n114 = call <vilib>:"WPI_SolenoidRefNum Registry Set.vi"("error in (no error)"=w91, "refnum name"=w93, "SolenoidDevRef"=w90) -> ("error out"=w89:errorcluster, "SolenoidDevRef"=w88:T23)  [unwired: 7 in]
  n115 = call-poly <vilib>:"WPI_CounterToDigitalSource.vi"("DigitalInputDevRef"=w34) -> ("Digital Source"=w32:T28)  [unwired: 6 out]
  n116 = call-poly <vilib>:"WPI_CounterToDigitalSource.vi"("DigitalInputDevRef"=w29) -> ("Digital Source"=w31:T28)  [unwired: 6 out]
  n117 = call-poly <vilib>:"WPI_CounterToDigitalSource.vi"("DigitalInputDevRef"=w41) -> ("Digital Source"=w43:T28)  [unwired: 6 out]
  n118 = call <vilib>:"WPI_SolenoidRefNum Registry Set.vi"("error in (no error)"=w96, "refnum name"=w94, "SolenoidDevRef"=w97) -> ("error out"=w98:errorcluster, "SolenoidDevRef"=w99:T23)  [unwired: 7 in]
  n119 = call <vilib>:"WPI_SwitchRefNum Registry Set.vi"("error in (no error)"=w64, "refnum name"=w67, "SwitchDevRef"=w63) -> ()  [unwired: 7 in, 2 out]
  n120 = call <vilib>:"WPI_EncoderOpen.vi"("BSource"=w51, "ASource"=w48) -> ("error out"=w47:errorcluster, "EncoderDevRef"=w46:T32)  [unwired: 6 in, 2 out]
  n121 = call-poly <vilib>:"WPI_CounterOpen.vi"("Up Source"=w11) -> ("error out"=w8:errorcluster, "CounterDevRef"=w10:T35)  [unwired: 6 in, 3 out]
  n122 = call <vilib>:"WPI_SwitchRefNum Registry Set.vi"("error in (no error)"=w69, "refnum name"=w72, "SwitchDevRef"=w68) -> ()  [unwired: 7 in, 2 out]
  n123 = call-poly <vilib>:"WPI_CounterOpen.vi"("Up Source"=w2) -> ("error out"=w5:errorcluster, "CounterDevRef"=w3:T35)  [unwired: 6 in, 3 out]
  n124 = call-poly <vilib>:"WPI_CounterOpen.vi"("Up Source"=w20) -> ("error out"=w24:errorcluster, "CounterDevRef"=w23:T35)  [unwired: 6 in, 3 out]
  n125 = call-poly <vilib>:"WPI_CounterOpen.vi"("Up Source"=w32) -> ("error out"=w36:errorcluster, "CounterDevRef"=w35:T35)  [unwired: 6 in, 3 out]
  n126 = call-poly <vilib>:"WPI_CounterOpen.vi"("Up Source"=w31) -> ("error out"=w27:errorcluster, "CounterDevRef"=w28:T35)  [unwired: 6 in, 3 out]
  n127 = call-poly <vilib>:"WPI_CounterOpen.vi"("Up Source"=w43) -> ("error out"=w39:errorcluster, "CounterDevRef"=w40:T35)  [unwired: 6 in, 3 out]
  n128 = call <vilib>:"WPI_EncoderRefNum Registry Set.vi"("error in (no error)"=w47, "refnum name"=w45, "EncoderDevRef"=w46) -> ()  [unwired: 7 in, 2 out]
  n129 = call <vilib>:"WPI_SolenoidSafetyConfig.vi"("error in (no error)"=w89, "mode"=WPI_SafetyOutputConfigMenu."Enable", "SolenoidDevRef"=w88) -> ()  [unwired: 7 in, 2 out]
  n130 = call <vilib>:"WPI_SolenoidSafetyConfig.vi"("error in (no error)"=w98, "mode"=WPI_SafetyOutputConfigMenu."Enable", "SolenoidDevRef"=w99) -> ()  [unwired: 7 in, 2 out]
  n131 = call <vilib>:"WPI_CounterRefNum Registry Set.vi"("error in (no error)"=w24, "refnum name"=w25, "CounterDevRef"=w23) -> ()  [unwired: 7 in, 2 out]
  n132 = call <vilib>:"WPI_CounterRefNum Registry Set.vi"("error in (no error)"=w36, "refnum name"=w37, "CounterDevRef"=w35) -> ()  [unwired: 7 in, 2 out]
  n133 = call <vilib>:"WPI_CounterRefNum Registry Set.vi"("error in (no error)"=w27, "refnum name"=w26, "CounterDevRef"=w28) -> ()  [unwired: 7 in, 2 out]
  n134 = call <vilib>:"WPI_CounterRefNum Registry Set.vi"("error in (no error)"=w8, "refnum name"=w7, "CounterDevRef"=w10) -> ()  [unwired: 7 in, 2 out]
  n135 = call <vilib>:"WPI_CounterRefNum Registry Set.vi"("error in (no error)"=w39, "refnum name"=w38, "CounterDevRef"=w40) -> ()  [unwired: 7 in, 2 out]
  n136 = call <vilib>:"WPI_CounterRefNum Registry Set.vi"("error in (no error)"=w5, "refnum name"=w6, "CounterDevRef"=w3) -> ()  [unwired: 7 in, 2 out]
  n137 = call-poly <vilib>:"WPI_SwitchOpen.vi"("DIO Channel"=FPGA_DIOChannel."DIO 5", "Controller"=FPGA_TypedefDigitalModule."Controller 1") -> ("error out"=w59:errorcluster, "SwitchDevRef"=w58:T24)  [unwired: 8 in]
  n138 = global read "Global Variables.vi" "Eject Encoder"() -> (w62:string)
  n139 = call <vilib>:"WPI_SwitchRefNum Registry Set.vi"("error in (no error)"=w59, "refnum name"=w62, "SwitchDevRef"=w58) -> ()  [unwired: 7 in, 2 out]
  n140 = global read "Global Variables.vi" "NavX"() -> (w13:string)
  n141 = call "navX Open.vi"("I2C Bus"=i2c_bus."I2C MXP", "SPI Bus"=spi_bus."SPI MXP", "Update Rate (4Hz-60Hz)"=T2 50, "navX Interface Protocol"=navX_Interface_Protocol."SPI") -> ("error out"=w15:errorcluster, "navX Device TypeDef"=w14:T36)  [unwired: 5 in, 1 out]
  n142 = global read "Global Variables.vi" "Joystick L 1"() -> (w216:string)
  n143 = call <vilib>:"WPI_JoystickOpen.vi"("JoystickDevice"=WPI_JoystickDeviceEnum."USB 2") -> ("JoystickDevRef"=w214:T45)  [unwired: 10 in]
  n144 = call <vilib>:"WPI_JoystickOpen.vi"("JoystickDevice"=WPI_JoystickDeviceEnum."USB 1") -> ("JoystickDevRef"=w217:T45)  [unwired: 10 in]
  n145 = global read "Global Variables.vi" "Joystick R 1"() -> (w213:string)
  n146 = call "navX SetRefnum.vi"("error in (no error)"=w15, "refnum name"=w13, "navX Device TypeDef"=w14) -> ()  [unwired: 7 in, 2 out]
  n147 = call <vilib>:"WPI_JoystickRefNum Registry Set.vi"("refnum name"=w213, "JoystickDevRef"=w214) -> ()  [unwired: 8 in, 2 out]
  n148 = call <vilib>:"WPI_JoystickRefNum Registry Set.vi"("refnum name"=w216, "JoystickDevRef"=w217) -> ()  [unwired: 8 in, 2 out]
